vi "create.vi"() -> ()   [LabVIEW 2013]
uses:
  <resource>/Framework/Providers/ws_project_provider/common/NI Web Service Provider.lvlib
panel:
  out "error out":errorcluster
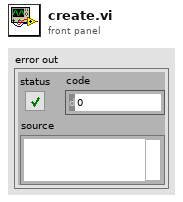
[diagram p1: front panel]
types:
  T1 = typedef "ws.ctl" = cluster{"Web Service":T2, "startup":path[], "wsmethods":path[], "private content":path[], "public content":path[], "wm ids":string[]}
  T2 = typedef "NI Web Service Provider.lvlib/Web Service.ctl" = cluster{"Name":string, "GUID":string, "Version":cluster{"Major":u16, "Minor":u16, "Fix":u16, "Build":u16}, "Serve index.html":bool, "Remote debugging":bool, "SSE2 optimizations":bool, "Exclusions":cluster{"Disconnect type definitions":bool, "Remove unused polymorphic VI instances":bool, "Remove unused members of project libraries":bool, "Modify project library file after removing unused members":bool}, "Disconnect inline subVIs":bool, "Auto-increment version":bool, "Web service VIs":T3[], "Static Permissions":string}
  T3 = typedef "NI Web Service Provider.lvlib/Web Service VI.ctl" = cluster{"item":u64, "item ID":string, "Web Service VI Type":T4, "Method":T5, "Load at startup":bool, "Keep in memory":bool, "Output type":T6, "Output format":T7, "Use headers":bool, "Buffered":bool, "Require API key":bool, "Permissions":string, "Standard URL":bool, "Include VI name in URL":bool, "Custom URL":string}
  T4 = typedef "NI Web Service Provider.lvlib/Web Service VI Type.ctl" = enum16{"<DUMMY>", "Web Method", "Auxiliary", "Internal", "Content"}
  T5 = typedef "NI Web Service Provider.lvlib/Web Service VI Method.ctl" = enum16{"<DUMMY>", "GET", "PUT", "POST", "DELETE", "OPTIONS", "HEAD", "TRACE"}
  T6 = typedef "NI Web Service Provider.lvlib/Web Service VI Output Type.ctl" = enum16{"Terminal", "Stream"}
  T7 = typedef "NI Web Service Provider.lvlib/Web Service VI Output Format.ctl" = enum16{"<DUMMY>", "Text", "XML", "HTML", "JSON"}
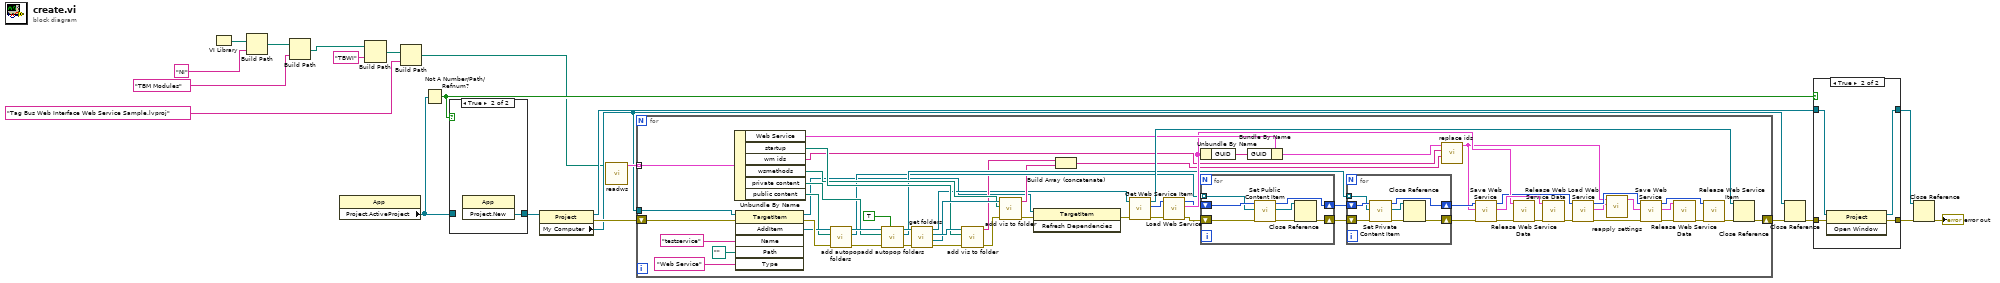
[diagram p0: block diagram]
diagram:
  n1 = VI Library() -> (path=w5:path)
  n2 = Build Path(base path=w5, name or relative path="NI") -> (appended path=w7:path)
  n3 = Build Path(base path=w7, name or relative path="TBM Modules") -> (appended path=w4:path)
  n4 = property class="App"() -> ("Project.ActiveProject"=w11:refnum<vi>)  [unwired: 2 in, 2 out]
  n5 = Build Path(base path=w4, name or relative path="TBWI") -> (appended path=w3:path)
  n6 = Build Path(base path=w3, name or relative path="Tag Bus Web Interface Web Service Sample.lvproj") -> (appended path=w1:path)
  n7 = Not A Number/Path/Refnum?(number/path/refnum=w11) -> (NaN/Path/Refnum?=w10:bool)
  n8 = case shown="True" w10 {
    tunnel: [w22 w23] -> w21
    tunnel: w11 -> [w22 _]
    frame False {
    }
    frame True {
      n9 = invoke class="App" method="Project.New"() -> ("Project:New"=w23:refnum<vi>)  [unwired: 3 in, 2 out]
    }
  }
  n10 = property class="Project"(reference=w21) -> (reference out=w17:refnum<vi>, error out=w19:errorcluster, "My Computer"=w13:refnum<vi>)  [unwired: 1 in]
  n11 = call "readws.vi"("Path"=w1) -> ("Array"=w20:T1[])  [unwired: 9 in, 1 out]
  n12 = for {
    tunnel: w20 -> [w65] mode=indexing
    shift-right: [w77] -> w12
    shift-left: w19 -> [w76]
    tunnel: w13 -> [w28]
    n13 = Unbundle By Name(w65) -> ("Web Service"=w60:T2, "startup"=w62:path[], "wm ids"=w43:string[], "wsmethods"=w61:path[], "private content"=w63:path[], "public content"=w64:path[])
    n14 = invoke class="TargetItem" method="AddItem"(reference=w28, error in=w76, "Name"="testservice", "Path"=path "", "Type"="Web Service") -> (reference out=w24:refnum<vi>, error out=w75:errorcluster, "AddItem"=w74:refnum<vi>)  [unwired: 1 in, 3 out]
    n15 = call "add autopop folders.vi"("error in (no error)"=w75, "autopop"=w64, "ProjectItem in"=w74) -> ("error out"=w69:errorcluster, "items out"=w46:refnum<vi>[], "ProjectItem out"=w66:refnum<vi>)  [unwired: 6 in]
    n16 = call "add autopop folders.vi"("private?"=TRUE, "error in (no error)"=w69, "autopop"=w63, "ProjectItem in"=w66) -> ("error out"=w68:errorcluster, "items out"=w47:refnum<vi>[], "ProjectItem out"=w67:refnum<vi>)  [unwired: 5 in]
    n17 = call "get folders.vi"("error in"=w68, "web service in"=w67) -> ("error out"=w72:errorcluster, "web methods"=w71:refnum<vi>, "startup"=w73:refnum<vi>, "Web service project item out"=w25:refnum<vi>)  [unwired: 6 in]
    n18 = call "add vis to folder.vi"("error in"=w72, "startup"=w62, "ProjectItem in"=w73) -> ("error out"=w70:errorcluster, "ids"=w40:string[])  [unwired: 7 in]
    n19 = call "add vis to folder.vi"("error in"=w70, "startup"=w61, "ProjectItem in"=w71) -> ("error out"=w27:errorcluster, "ids"=w42:string[])  [unwired: 7 in]
    n20 = invoke class="TargetItem" method="Refresh Dependencies"(reference=w24, error in=w27) -> (error out=w26:errorcluster)  [unwired: 1 in, 2 out]
    n21 = Build Array (concatenate)(w40, w42) -> (w41:string[])
    n22 = call <resource>:"Get Web Service Item.vi"("Error In"=w26, "Web service project item"=w25) -> ("Error Out"=w58:errorcluster, "Web service item"=w59:u64, "Web service project item out"=w78:refnum<vi>)  [unwired: 7 in]
    n23 = call <resource>:"Load Web Service.vi"("Error In"=w58, "Web service item"=w59) -> ("Error Out"=w52:errorcluster, "Web Service"=w54:T2, "Web service item out"=w49:u64)  [unwired: 7 in]
    n24 = Unbundle By Name(w54) -> ("GUID"=w57:string)
    n25 = for {
      shift-right: [w91] -> w44
      shift-left: w52 -> [w94]
      shift-right: [w97] -> w50
      shift-left: w49 -> [w93]
      tunnel: w46 -> [w92] mode=indexing
      n26 = call <resource>:"Set Public Content Item.vi"("Error In"=w94, "Public content project item"=w92, "Web service item"=w93) -> ("Error Out"=w96:errorcluster, "Public content project item out"=w95:refnum<vi>, "Web service item out"=w97:u64)  [unwired: 6 in]
      n27 = Close Reference(reference=w95, error in (no error)=w96) -> (error out=w91:errorcluster)
    }
    n28 = Bundle By Name(cluster=w60, "GUID"=w57) -> (w45:T2)
    n29 = for {
      shift-right: [w90] -> w51
      shift-left: w44 -> [w85]
      shift-right: [w88] -> w48
      shift-left: w50 -> [w89]
      tunnel: w47 -> [w84] mode=indexing
      n30 = call <resource>:"Set Private Content Item.vi"("Error In"=w85, "Private content project item"=w84, "Web service item"=w89) -> ("Error Out"=w86:errorcluster, "Private content project item out"=w87:refnum<vi>, "Web service item out"=w88:u64)  [unwired: 6 in]
      n31 = Close Reference(reference=w87, error in (no error)=w86) -> (error out=w90:errorcluster)
    }
    n32 = call "replace ids.vi"("new ids"=w41, "old ids"=w43, "Web Service in"=w45) -> ("Web Service out"=w31:T2)  [unwired: 8 in]
    n33 = call <resource>:"Save Web Service.vi"("Error In"=w51, "Web Service"=w31, "Web service item"=w48) -> ("Error Out"=w56:errorcluster, "Web Service out"=w80:T2, "Web service item out"=w39:u64)  [unwired: 6 in]
    n34 = call <resource>:"Release Web Service Data.vi"("Error In"=w56, "Web Service"=w54) -> ("Error Out"=w55:errorcluster)  [unwired: 9 in]
    n35 = call <resource>:"Release Web Service Data.vi"("Error In"=w55, "Web Service"=w80) -> ("Error Out"=w38:errorcluster)  [unwired: 9 in]
    n36 = call <resource>:"Load Web Service.vi"("Error In"=w38, "Web service item"=w39) -> ("Error Out"=w32:errorcluster, "Web Service"=w29:T2, "Web service item out"=w34:u64)  [unwired: 7 in]
    n37 = call "reapply settings.vi"("ws settings in"=w29, "desired settings"=w31) -> ("ws settings out"=w30:T2)  [unwired: 9 in]
    n38 = call <resource>:"Save Web Service.vi"("Error In"=w32, "Web Service"=w30, "Web service item"=w34) -> ("Error Out"=w37:errorcluster, "Web Service out"=w33:T2, "Web service item out"=w35:u64)  [unwired: 6 in]
    n39 = call <resource>:"Release Web Service Data.vi"("Error In"=w37, "Web Service"=w33) -> ("Error Out"=w36:errorcluster)  [unwired: 9 in]
    n40 = call <resource>:"Release Web Service Item.vi"("Error In"=w36, "Web service item"=w35) -> ("Error Out"=w79:errorcluster)  [unwired: 9 in]
    n41 = Close Reference(reference=w78, error in (no error)=w79) -> (error out=w77:errorcluster)
  }
  n42 = Close Reference(reference=w13, error in (no error)=w12) -> (error out=w18:errorcluster)
  n43 = case shown="True" w10 {
    tunnel: w18 -> [w98 w103]
    tunnel: w17 -> [w99 w102]
    tunnel: [w98 w101] -> w16
    tunnel: [w99 w100] -> w15
    frame False {
    }
    frame True {
      n44 = invoke class="Project" method="Open Window"(reference=w102, error in=w103) -> (reference out=w100:refnum<vi>, error out=w101:errorcluster)  [unwired: 1 in, 1 out]
    }
  }
  n45 = Close Reference(reference=w15, error in (no error)=w16) -> (error out=→"error out":errorcluster)
